vi "DataTreeCtrl refreshFileTree.vi"(8 "error in (no error)":errorcluster, 11 "DataTreeCtrl in":refnum<class "DataTreeCtrl.lvclass">) -> (0 "error out":errorcluster, 3 "DataTreeCtrl out":refnum<class "DataTreeCtrl.lvclass">)   [LabVIEW 2018, in "DataTreeCtrl.lvclass"]
uses:
  DataTreeCtrl.lvclass
  DataTreeCtrl.lvclass/DataTreeCtrl.ctl
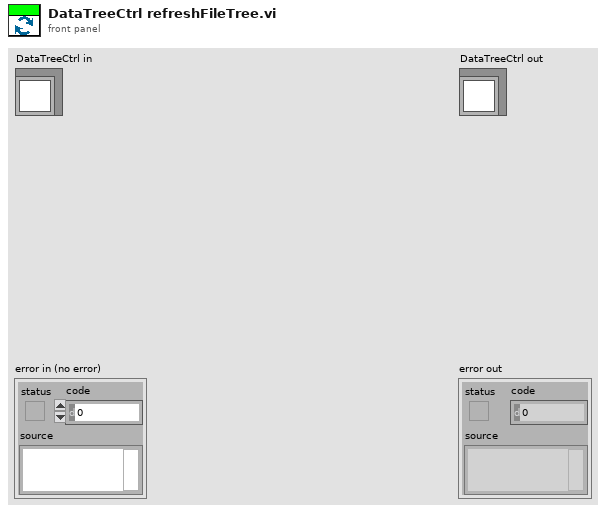
[diagram p1: front panel]
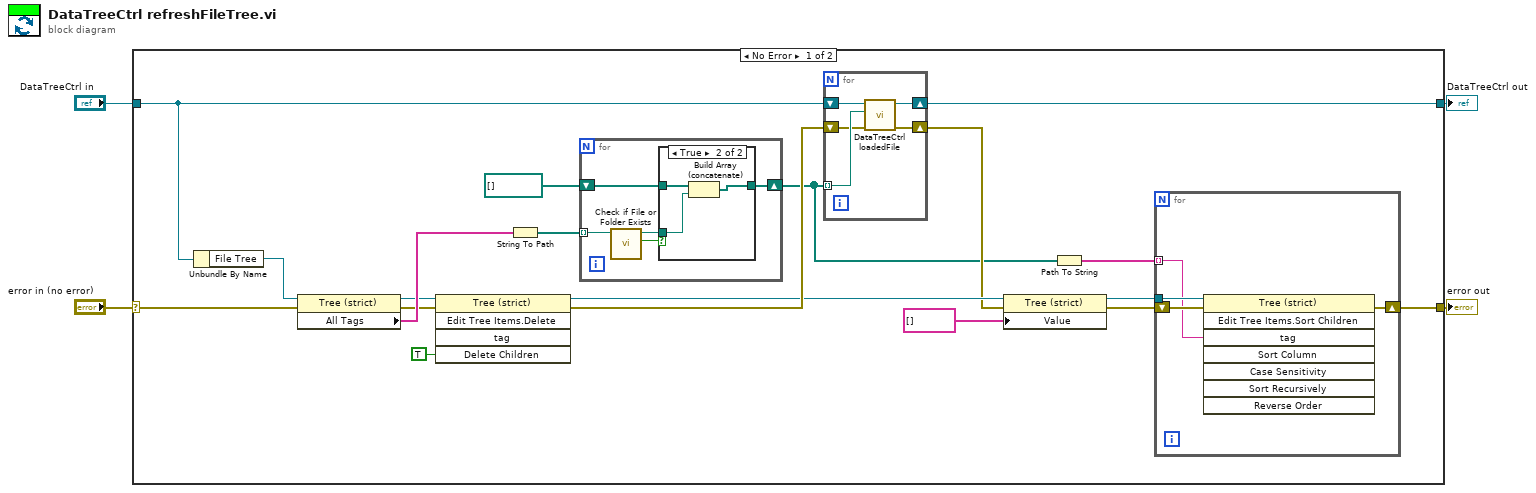
[diagram p0: block diagram]
diagram:
  n1 = case shown="No Error" "error in (no error)" {
    selector: "error in (no error)" -> [w17 w43]
    tunnel: [w7 w43] -> w3
    tunnel: [w13 w42] -> w1
    tunnel: "DataTreeCtrl in" -> [w15 w42]
    frame No Error {
      n2 = Unbundle By Name(w15) -> ("File Tree"=w16:refnum<vi>)
      n3 = property class="Tree (strict)"(reference=w16, error in=w17) -> (reference out=w19:refnum<vi>, error out=w18:errorcluster, "All Tags"=w23:string[])
      n4 = invoke class="Tree (strict)" method="Edit Tree Items.Delete"(reference=w19, error in=w18, "Delete Children"=TRUE ("Delete Children?")) -> (reference out=w12:refnum<vi>, error out=w14:errorcluster)  [unwired: 2 in, 3 out]
      n5 = String To Path(string=w23) -> (path=w22:path[])
      n6 = for {
        tunnel: w22 -> [w37] mode=indexing
        shift-right: [w33] -> w6
        shift-left: path[] [] -> [w35]
        n7 = call <vilib>:"Check if File or Folder Exists.vi"("path"=w37) -> ("file or folder exists?"=w36:bool, "dup path"=w34:path)  [unwired: 8 in, 1 out]
        n8 = case shown="True" w36 {
          tunnel: w35 -> [w38 w41]
          tunnel: w34 -> [_ w40]
          tunnel: [w38 w39] -> w33
          frame False {
          }
          frame True {
            n9 = Build Array (concatenate)(w41, w40) -> (w39:path[])
          }
        }
      }
      n10 = for {
        shift-right: [w32] -> w13
        shift-left: w15 -> [w31]
        tunnel: w6 -> [w30] mode=indexing
        shift-right: [w28] -> w11
        shift-left: w14 -> [w29]
        n11 = call "DataTreeCtrl loadedFile.vi"("error in (no error)"=w29, "filePath"=w30, "DataTreeCtrl in"=w31) -> ("error out"=w28:errorcluster, "DataTreeCtrl out"=w32:refnum<class "DataTreeCtrl.lvclass">)  [unwired: 7 in]
      }
      n12 = property class="Tree (strict)"(reference=w12, error in=w11, "Value"=string[] []) -> (reference out=w9:refnum<vi>, error out=w8:errorcluster)
      n13 = Path To String(path=w6) -> (string=w5:string[])
      n14 = for {
        tunnel: w9 -> [w27]
        shift-right: [w25] -> w7
        shift-left: w8 -> [w26]
        tunnel: w5 -> [w24] mode=indexing
        n15 = invoke class="Tree (strict)" method="Edit Tree Items.Sort Children"(reference=w27, error in=w26, "tag"=w24) -> (error out=w25:errorcluster)  [unwired: 5 in, 7 out]
      }
    }
    frame Error {
    }
  }
  "error out" <- w3
  "DataTreeCtrl out" <- w1
